vi "Write Snippet.vi"(8 "error in (no error)":errorcluster, 10 "VI Snippet (.png)":path, 11 "Snippet":T1) -> (0 "error out":errorcluster)   [LabVIEW 2022 SP3, in "VI-Snippet.lvlib"]
doc: "Writes a VI Snippet image and embeds the VI."
uses:
  VI-Snippet.lvlib
  Snippet.ctl
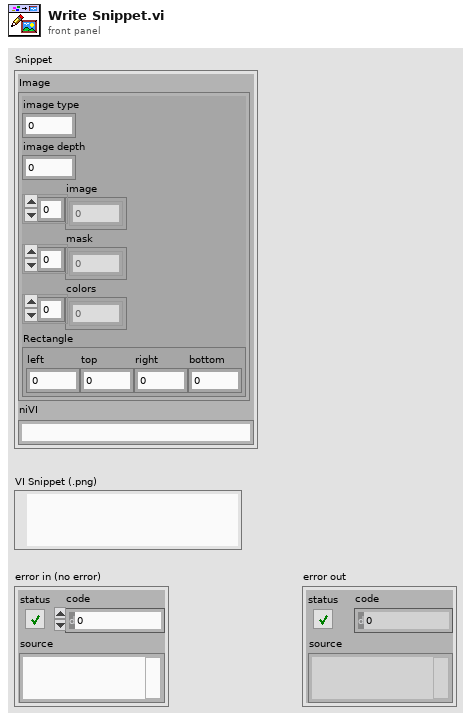
[diagram p1: front panel]
types:
  T1 = typedef "VI-Snippet.lvlib/Snippet.ctl" = cluster{"Image":cluster{"image type":i32, "image depth":i32, "image":u8[], "mask":u8[], "colors":u32[], "Rectangle":cluster{"left":i16, "top":i16, "right":i16, "bottom":i16}}, "niVI":string}
  T2 = cluster{"image type":i32, "image depth":i32, "image":u8[], "mask":u8[], "colors":u32[], "Rectangle":cluster{"left":i16, "top":i16, "right":i16, "bottom":i16}}
  T3 = cluster{"Length":i32, "Type":string, "Data":string, "CRC":u32}
  T4 = cluster{"Length":i32, "Type":string, "Data":string, "CRC":u32}[]
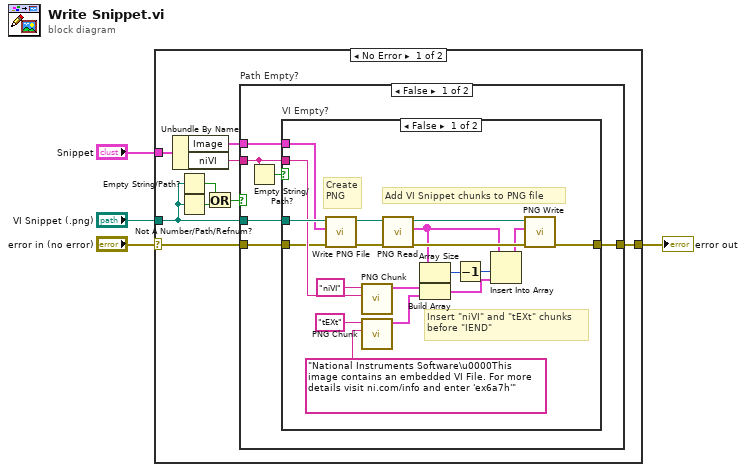
[diagram p0: block diagram]
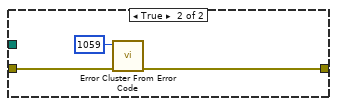
[diagram p2: hidden frame]
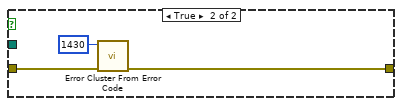
[diagram p3: hidden frame]
diagram:
  n1 = case shown="No Error" "error in (no error)" {
    selector: "error in (no error)" -> [w13 w45]
    tunnel: "Snippet" -> [w5 _]
    tunnel: [w12 w45] -> w3
    tunnel: "VI Snippet (.png)" -> [w6 _]
    frame No Error {
      n2 = Unbundle By Name(w5) -> ("Image"=w7:T2, "niVI"=w8:string)
      n3 = Empty String/Path?(string/path=w6) -> (empty?=w10:bool)
      n4 = Not A Number/Path/Refnum?(number/path/refnum=w6) -> (NaN/Path/Refnum?=w11:bool)
      n5 = Or(x=w10, y=w11) -> (x .or. y?=w9:bool)
      n6 = case "Path Empty?" shown="False" w9 {
        tunnel: w13 -> [w16 w44]
        tunnel: w6 -> [w19 _]
        tunnel: w7 -> [w18 _]
        tunnel: [w17 w42] -> w12
        tunnel: w8 -> [w15 _]
        frame False {
          n7 = Empty String/Path?(string/path=w15) -> (empty?=w14:bool)
          n8 = case "VI Empty?" shown="False" w14 {
            tunnel: w19 -> [w38 _]
            tunnel: w18 -> [w37 _]
            tunnel: [w26 w39] -> w17
            tunnel: w15 -> [w21 _]
            tunnel: w16 -> [w20 w40]
            frame False {
              # "Create\nPNG"
              # "Add VI Snippet chunks to PNG file"
              # "Insert \"niVI\" and \"tEXt\" chunks\nbefore \"IEND\""
              n9 = call <vilib>:"Write PNG File.vi"("error in (no error)"=w20, "image data"=w37, "path to PNG file"=w38) -> ("error out"=w22:errorcluster, "path"=w25:path)  [unwired: 7 in]
              n10 = call "PNG Chunk.vi"("Data"=w21, "Type"="niVI") -> ("PNG Chunk"=w29:T3)  [unwired: 9 in]
              n11 = call "PNG Chunk.vi"("Data"="National Instruments Software\u0000This image contains an embedded VI File. For more details visit ni.com/info and enter 'ex6a7h'", "Type"="tEXt") -> ("PNG Chunk"=w28:T3)  [unwired: 9 in]
              n12 = call "PNG Read.vi"("error in (no error)"=w22, "Image Path (*.png)"=w25) -> ("error out"=w36:errorcluster, "Chunks"=w24:T4, "dup Image Path"=w23:path)  [unwired: 7 in]
              n13 = Array Size(array=w24) -> (size(s)=w34:i32)
              n14 = Build Array(w29, w28) -> (w27:T4)
              n15 = Decrement(x=w34) -> (x-1=w33:i32)
              n16 = Insert Into Array(array=w24, index=w33, new element=w27) -> (w35:T4)
              n17 = call "PNG Write.vi"("error in (no error)"=w36, "Chunks"=w35, "Image Path (*.png)"=w23) -> ("error out"=w26:errorcluster)  [unwired: 7 in, 1 out]
            }
            frame True {
              n18 = call <vilib>:"Error Cluster From Error Code.vi"("error in (no error)"=w40, "error code (0)"=1059 ("code")) -> ("error out"=w39:errorcluster)  [unwired: 7 in]
            }
          }
        }
        frame True {
          n19 = call <vilib>:"Error Cluster From Error Code.vi"("error in (no error)"=w44, "error code (0)"=1430 ("code")) -> ("error out"=w42:errorcluster)  [unwired: 7 in]
        }
      }
    }
    frame Error {
    }
  }
  "error out" <- w3
